vi "首页显示设置.vi"() -> ()   [LabVIEW 2016]
uses:
  <vilib>/Utility/miscctls.llb/LVPointTypeDef.ctl
  <vilib>/Utility/config.llb/NI_LVConfig.lvlib
panel:
  in  "磷酸盐":bool caption="氨氮禁用"
  in  "CODCr":bool caption="氨氮禁用"
  in  "ORP":bool caption="氨氮禁用"
  in  "硫化物":bool caption="氨氮禁用"
  in  "亚硝氮":bool caption="氨氮禁用"
  in  "硝氮":bool caption="氨氮禁用"
  in  "确认":bool
  in  "藻密度":bool=TRUE caption="氨氮禁用"
  in  "叶绿素a":bool=TRUE caption="氨氮禁用"
  in  "湿度":bool=TRUE caption="氨氮禁用"
  in  "室温":bool=TRUE caption="氨氮禁用"
  in  "电压":bool=TRUE caption="氨氮禁用"
  in  "CODMn":bool=TRUE caption="氨氮禁用"
  in  "总氮":bool=TRUE caption="氨氮禁用"
  in  "总磷":bool=TRUE caption="氨氮禁用"
  in  "氨氮":bool=TRUE caption="氨氮禁用"
  in  "Turb":bool=TRUE caption="氨氮禁用"
  in  "Cond":bool=TRUE caption="氨氮禁用"
  in  "DO":bool=TRUE caption="氨氮禁用"
  in  "pH":bool=TRUE caption="氨氮禁用"
  in  "水温":bool=TRUE caption="氨氮禁用"
  # "请选择首页要显示的参数"
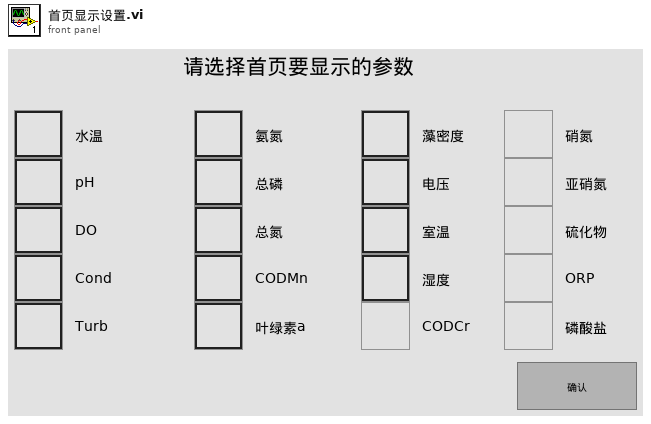
[diagram p1: front panel]
types:
  T1 = typedef "LVPointTypeDef.ctl" = cluster{"Horizontal":i16, "Vertical":i16}
  T2 = typedef "NI_LVConfig.lvlib/Config Data RefNum.ctl" = refnum<k1>
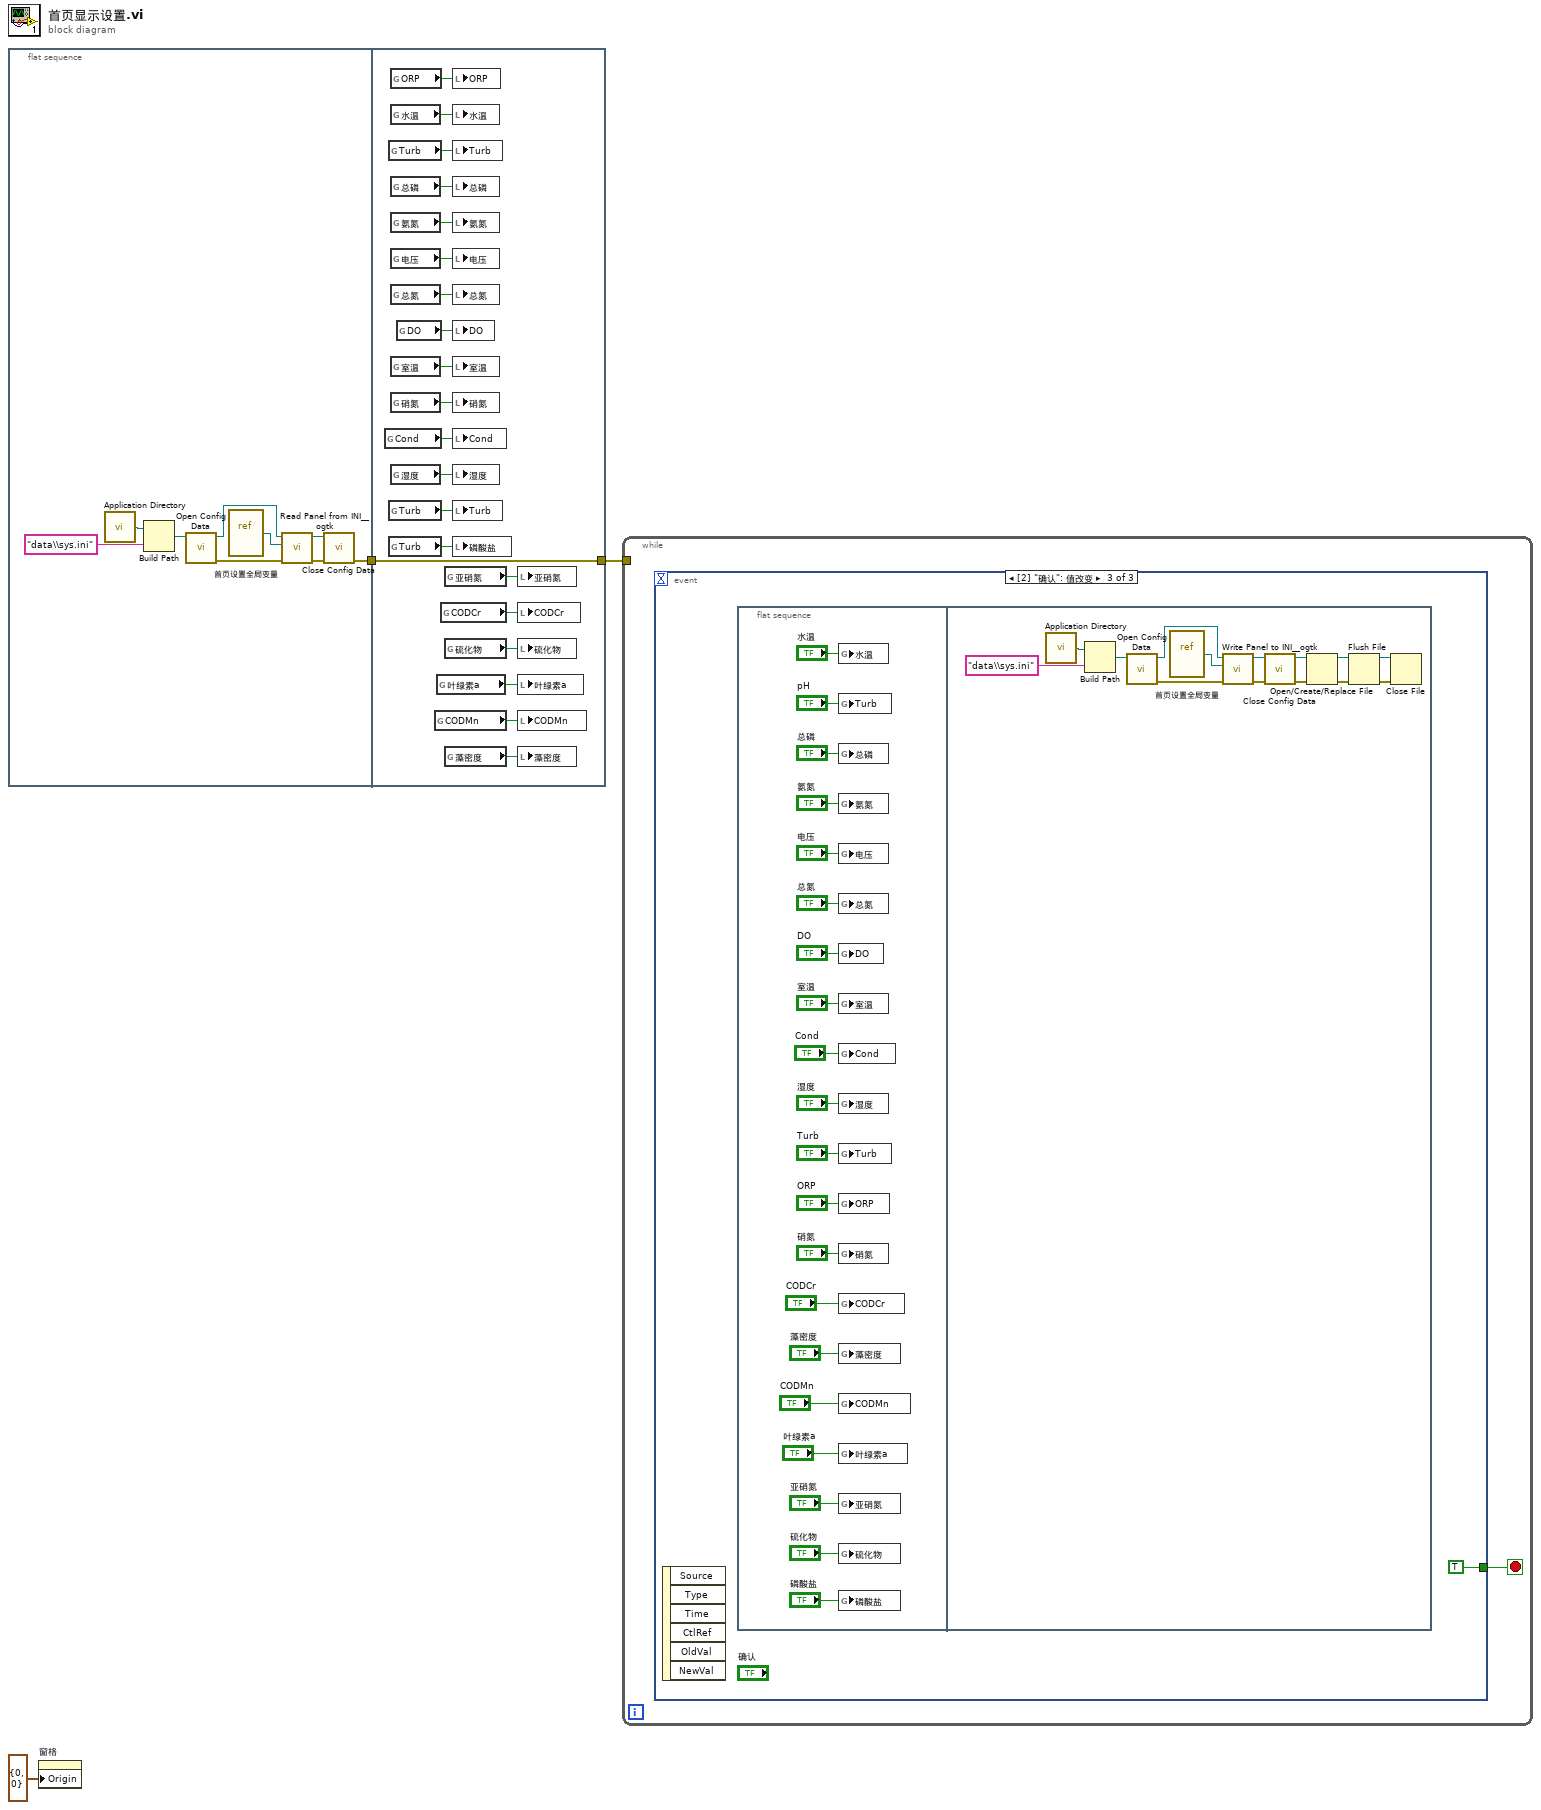
[diagram p0: block diagram]
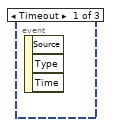
[diagram p2: hidden frame]
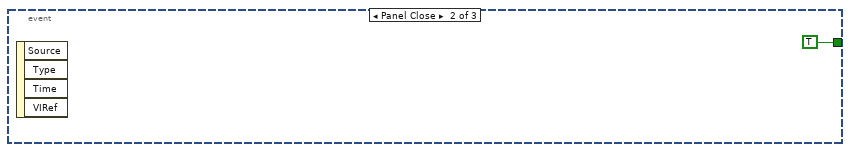
[diagram p3: hidden frame]
diagram:
  n1 = flat-sequence {
    tunnel: [w4] -> w2
    tunnel: w2 -> [w19]
    tunnel: [w19] -> w1
    frame #0 {
      n2 = call <vilib>:"Application Directory.vi"() -> ("Application Directory"=w12:path)
      n3 = Build Path(base path=w12, name or relative path="data\\sys.ini" ("名称或相对路径")) -> (appended path=w10:path)
      n4 = call <vilib>:"Open Config Data.vi"("configuration file path"=w10) -> ("error out"=w6:errorcluster, "refnum"=w9:T2)  [unwired: 8 in, 1 out]
      n5 = vi-ref "首页设置全局变量.vi"() -> (w8:refnum<vi>)
      n6 = call <userlib>:"Read Panel from INI__ogtk.vi"("error in (no error)"=w6, "VI ref"=w8, "refnum"=w9) -> ("error out"=w5:errorcluster, "refnum out"=w7:T2)  [unwired: 7 in]
      n7 = call <vilib>:"Close Config Data.vi"("error in (no error)"=w5, "refnum"=w7) -> ("error out"=w4:errorcluster)  [unwired: 8 in, 1 out]
    }
    frame #1 {
      n8 = global read "首页设置全局变量.vi" "Cond"() -> (w20:bool)
      n9 = global read "首页设置全局变量.vi" "Turb"() -> (w27:bool)
      n10 = global read "首页设置全局变量.vi" "Turb"() -> (w29:bool)
      n11 = global read "首页设置全局变量.vi" "Turb"() -> (w13:bool)
      n12 = global read "首页设置全局变量.vi" "ORP"() -> (w15:bool)
      n13 = global read "首页设置全局变量.vi" "水温"() -> (w28:bool)
      n14 = global read "首页设置全局变量.vi" "总磷"() -> (w26:bool)
      n15 = global read "首页设置全局变量.vi" "氨氮"() -> (w25:bool)
      n16 = global read "首页设置全局变量.vi" "电压"() -> (w24:bool)
      n17 = global read "首页设置全局变量.vi" "总氮"() -> (w23:bool)
      n18 = global read "首页设置全局变量.vi" "室温"() -> (w21:bool)
      n19 = global read "首页设置全局变量.vi" "硝氮"() -> (w18:bool)
      n20 = global read "首页设置全局变量.vi" "湿度"() -> (w33:bool)
      n21 = global read "首页设置全局变量.vi" "DO"() -> (w22:bool)
      n22 = global read "首页设置全局变量.vi" "CODMn"() -> (w31:bool)
      n23 = global read "首页设置全局变量.vi" "叶绿素a"() -> (w30:bool)
      n24 = global read "首页设置全局变量.vi" "CODCr"() -> (w14:bool)
      n25 = global read "首页设置全局变量.vi" "亚硝氮"() -> (w17:bool)
      n26 = global read "首页设置全局变量.vi" "硫化物"() -> (w16:bool)
      n27 = global read "首页设置全局变量.vi" "藻密度"() -> (w32:bool)
      n28 = local write "ORP"(w15) -> ()
      n29 = local write "水温"(w28) -> ()
      n30 = local write "Turb"(w27) -> ()
      n31 = local write "总磷"(w26) -> ()
      n32 = local write "氨氮"(w25) -> ()
      n33 = local write "电压"(w24) -> ()
      n34 = local write "总氮"(w23) -> ()
      n35 = local write "DO"(w22) -> ()
      n36 = local write "室温"(w21) -> ()
      n37 = local write "硝氮"(w18) -> ()
      n38 = local write "Cond"(w20) -> ()
      n39 = local write "湿度"(w33) -> ()
      n40 = local write "Turb"(w29) -> ()
      n41 = local write "磷酸盐"(w13) -> ()
      n42 = local write "亚硝氮"(w17) -> ()
      n43 = local write "CODCr"(w14) -> ()
      n44 = local write "硫化物"(w16) -> ()
      n45 = local write "叶绿素a"(w30) -> ()
      n46 = local write "CODMn"(w31) -> ()
      n47 = local write "藻密度"(w32) -> ()
    }
  }
  n48 = property on="窗格" class="Pane"("Origin"=T1 {"Horizontal"=0, "Vertical"=0} ("原点")) -> ()  [unwired: 2 in, 2 out]
  n49 = while {
    tunnel: w1 -> [_]
    stop <- w34 stop-if-true
    n50 = event shown="[2] \"确认\": 值改变" {
      selector: _ -> [_ _ _]
      dyn-events: _ -> [_ _ _]
      timeout: _ -> [_ _ _]
      tunnel: [_ TRUE TRUE] -> w34
      event Timeout {
        n51 = event-data() -> ()  [unwired: 1 in, 3 out]
      }
      event Panel Close {
        n52 = event-data() -> ()  [unwired: 1 in, 4 out]
      }
      event "确认": Value Change {
        n53 = event-data() -> ()  [unwired: 1 in, 6 out]
        n54 = flat-sequence {
          frame #0 {
            n55 = global write "首页设置全局变量.vi" "水温"("水温") -> ()
            n56 = global write "首页设置全局变量.vi" "Turb"("pH") -> ()
            n57 = global write "首页设置全局变量.vi" "总磷"("总磷") -> ()
            n58 = global write "首页设置全局变量.vi" "氨氮"("氨氮") -> ()
            n59 = global write "首页设置全局变量.vi" "电压"("电压") -> ()
            n60 = global write "首页设置全局变量.vi" "总氮"("总氮") -> ()
            n61 = global write "首页设置全局变量.vi" "DO"("DO") -> ()
            n62 = global write "首页设置全局变量.vi" "室温"("室温") -> ()
            n63 = global write "首页设置全局变量.vi" "Cond"("Cond") -> ()
            n64 = global write "首页设置全局变量.vi" "湿度"("湿度") -> ()
            n65 = global write "首页设置全局变量.vi" "Turb"("Turb") -> ()
            n66 = global write "首页设置全局变量.vi" "ORP"("ORP") -> ()
            n67 = global write "首页设置全局变量.vi" "硝氮"("硝氮") -> ()
            n68 = global write "首页设置全局变量.vi" "CODCr"("CODCr") -> ()
            n69 = global write "首页设置全局变量.vi" "藻密度"("藻密度") -> ()
            n70 = global write "首页设置全局变量.vi" "CODMn"("CODMn") -> ()
            n71 = global write "首页设置全局变量.vi" "叶绿素a"("叶绿素a") -> ()
            n72 = global write "首页设置全局变量.vi" "亚硝氮"("亚硝氮") -> ()
            n73 = global write "首页设置全局变量.vi" "硫化物"("硫化物") -> ()
            n74 = global write "首页设置全局变量.vi" "磷酸盐"("磷酸盐") -> ()
          }
          frame #1 {
            n75 = call <vilib>:"Application Directory.vi"() -> ("Application Directory"=w57:path)
            n76 = Build Path(base path=w57, name or relative path="data\\sys.ini" ("名称或相对路径")) -> (appended path=w59:path)
            n77 = call <vilib>:"Open Config Data.vi"("configuration file path"=w59) -> ("error out"=w63:errorcluster, "refnum"=w60:T2)  [unwired: 8 in, 1 out]
            n78 = vi-ref "首页设置全局变量.vi"() -> (w61:refnum<vi>)
            n79 = call <userlib>:"Write Panel to INI__ogtk.vi"("error in (no error)"=w63, "VI ref"=w61, "refnum"=w60) -> ("error out"=w64:errorcluster, "refnum out"=w62:T2)  [unwired: 7 in]
            n80 = call <vilib>:"Close Config Data.vi"("error in (no error)"=w64, "refnum"=w62) -> ("error out"=w69:errorcluster, "file path"=w70:path)  [unwired: 8 in]
            n81 = Open/Create/Replace File(file path (use dialog)=w70, error in=w69) -> (refnum out=w66:refnum<file>, error out=w65:errorcluster)  [unwired: 4 in, 1 out]
            n82 = Flush File(refnum=w66, error in=w65) -> (refnum out=w67:refnum<file>, error out=w68:errorcluster)
            n83 = Close File(refnum=w67, error in=w68) -> ()  [unwired: 2 out]
          }
        }
      }
    }
  }
